vi "Fire User Event - Stop.vi"(8 "error in (no error)":errorcluster caption="错误输入（无错误）", 11 "User Event - Stop":refnum<user-event> caption="用户事件－停止") -> (0 "error out":errorcluster caption="错误输出")   [LabVIEW 2013, in "User Event - Stop.lvlib"]
doc: "发送“停止”事件的对应消息，使“事件处理循环”停止运行。"
uses:
  User Event - Stop.lvlib
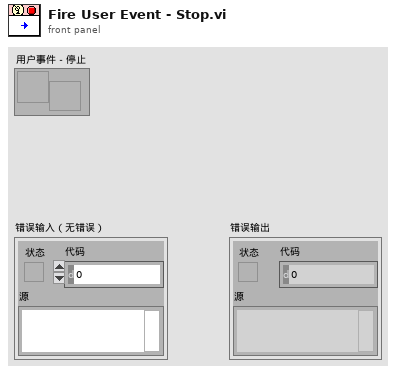
[diagram p1: front panel]
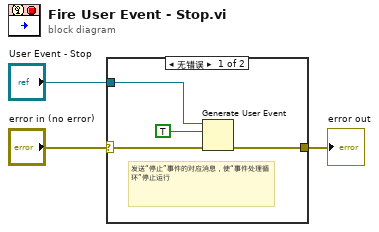
[diagram p0: block diagram]
diagram:
  n1 = case shown="无错误" "error in (no error)" {
    selector: "error in (no error)" -> [w4 w8]
    tunnel: [w6 w8] -> w3
    tunnel: "User Event - Stop" -> [w5 _]
    frame No Error {
      # "发送“停止”事件的对应消息，使“事件处理循环”停止运行"
      n2 = Generate User Event(user event=w5, event data cluster=TRUE ("event data"), error in=w4) -> (error out=w6:errorcluster)  [unwired: 1 in, 1 out]
    }
    frame Error {
    }
  }
  "error out" <- w3
